vi "Split Registers by Direction.vi"(8 "error in":errorcluster, 11 "vi info":T1 {"RegisterMap"."Address" format="%.0x"}) -> (0 "error out":errorcluster, 2 "Controls":T8[](array[typedef]) {"Data Type" format="%.0x"}, 3 "Indicator":T8[](array[typedef]) {"Data Type" format="%.0x"})   [LabVIEW 2016, in "FPGA Addon System Explorer.lvlib"]
uses:
  FPGA Addon System Explorer.lvlib
  Shared/Register Information.ctl
  Shared/Data Type.ctl
  <vilib>/rvi/Bitfile/niFpgaBitfileStructure_VI.ctl
  <vilib>/rvi/Bitfile/nirviControlStructure.ctl
  <vilib>/rvi/Bitfile/nirviTypdefDescription.ctl
  <vilib>/rvi/Bitfile/nirviMechanicalAction.ctl
  <vilib>/rvi/Bitfile/nirviSubControlStructure.ctl
  <vilib>/rvi/Bitfile/nirviClusterElementControl.ctl
  <vilib>/picture/picture.llb/imagedata.ctl
  FPGA/Speciality IO/Types/PWM.Measure.Analog.Measurement.ctl
  FPGA/Speciality IO/Types/PWM.Measure.Digital.Measurement.ctl
  FPGA/Speciality IO/Types/PWM.Generate.Digital.Settings.ctl
  FPGA/Speciality IO/Types/PWM.Measure.Analog.Settings.ctl
  FPGA/Speciality IO/Types/PWM.Measure.Digital.Settings.ctl
  FPGA/Speciality IO/Types/Sine.Generate.Settings.ctl
  Shared/FPGA Addon Shared.lvlib
  FPGA/Speciality IO/Speciality FPGA IO.lvlib
  <vilib>/Utility/Data Type/NI_Data Type.lvlib
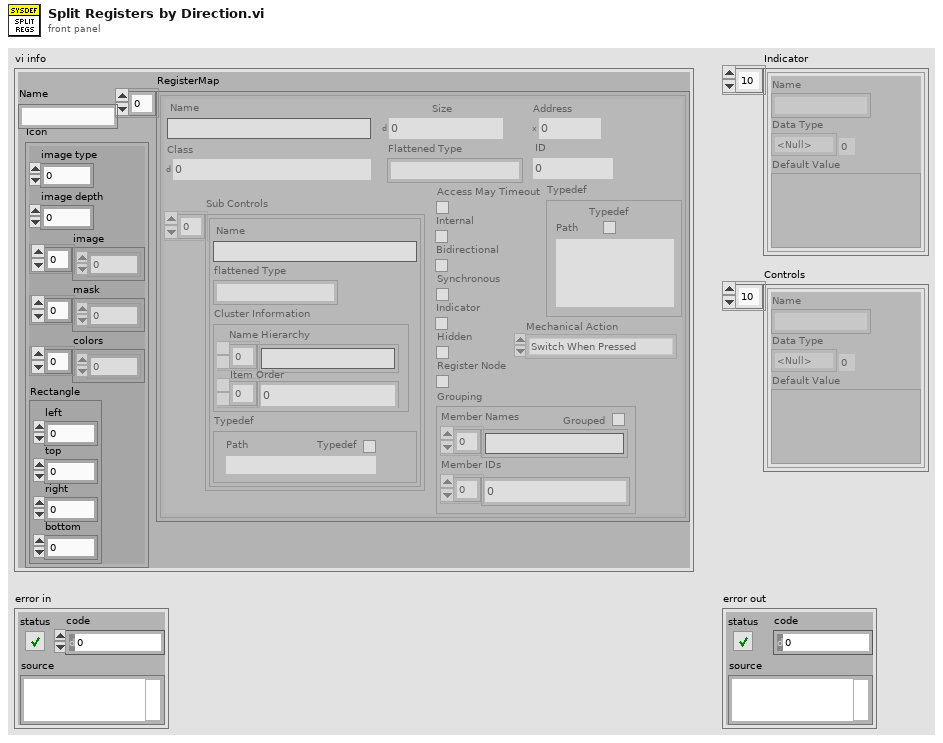
[diagram p1: front panel]
types:
  T1 = typedef "niFpgaBitfileStructure_VI.ctl" = cluster{"Name":string, "RegisterMap":T2[], "Icon":T7}
  T2 = typedef "nirviControlStructure.ctl" = cluster{"Name":string, "Hidden":bool, "Indicator":bool, "Flattened Type":string, "Grouping":cluster{"Grouped":bool, "Member Names":string[], "Member IDs":u32[]}, "Address":u32, "Size":u32, "Class":u32, "Internal":bool, "Typedef":T3, "ID":u32, "Bidirectional":bool, "Synchronous":bool, "Mechanical Action":T4, "Sub Controls":T5[], "Access May Timeout":bool, "Register Node":bool}
  T3 = typedef "nirviTypdefDescription.ctl" = cluster{"Typedef":bool, "Path":path}
  T4 = typedef "nirviMechanicalAction.ctl" = enum8{"Switch When Pressed", "Switch When Released", "Switch Until Released", "Latch When Pressed", "Latch When Released", "Latch Until Released"}
  T5 = typedef "nirviSubControlStructure.ctl" = cluster{"Name":string, "flattened Type":string, "Cluster Information":T6, "Typedef":T3}
  T6 = typedef "nirviClusterElementControl.ctl" = cluster{"Name Hierarchy":string[], "Item Order":u32[]}
  T7 = typedef "imagedata.ctl" = cluster{"image type":i32, "image depth":i32, "image":u8[], "mask":u8[], "colors":u32[], "Rectangle":cluster{"left":i16, "top":i16, "right":i16, "bottom":i16}}
  T8 = typedef "FPGA Addon Shared.lvlib/Register Information.ctl" = cluster{"Name":string, "Data Type":T9, "Default Value":variant}
  T9 = typedef "FPGA Addon Shared.lvlib/Data Type.ctl" = enum8{"<Null>", "I8", "I16", "I32", "I64", "U8", "U16", "U32", "U64", "SGL", "Boolean", "Analog PWM In Settings", "Analog PWM In", "Digital PWM In Settings", "Digital PWM In", "Digital PWM Out", "Sine Out", "FXP+/-24.5", "FXP+/-16.5", "FXP+/-32.8", "FXP+/-64.32", "FXP+/-16.7", "FXP+/-20.5"}
  T10 = typedef "Speciality FPGA IO.lvlib/PWM.Measure.Digital.Measurement.ctl" = cluster{"ACTIVE TICKS":u32, "INACTIVE TICKS":u32, "ACQ TICKS":u32}
  T11 = typedef "Speciality FPGA IO.lvlib/PWM.Measure.Analog.Measurement.ctl" = cluster{"ACTIVE TICKS":u32, "INACTIVE TICKS":u32, "ACQ TICKS":u32, "ACTIVE VOLTAGE":fxp<+/-,32,8>, "INACTIVE VOLTAGE":fxp<+/-,32,8>}
  T12 = typedef "Speciality FPGA IO.lvlib/Sine.Generate.Settings.ctl" = cluster{"AMP":fxp<+/-,32,8>, "OFFSET":fxp<+/-,32,8>, "PERIODS/TICKS":fxp<+,32,0>}
  T13 = typedef "Speciality FPGA IO.lvlib/PWM.Measure.Digital.Settings.ctl" = cluster{"ACTIVE EDGE":bool, "TIMEOUT":u32}
  T14 = typedef "Speciality FPGA IO.lvlib/PWM.Measure.Analog.Settings.ctl" = cluster{"ACTIVE EDGE":bool, "TIMEOUT":u32, "THRESHOLD":fxp<+/-,32,8>}
  T15 = typedef "Speciality FPGA IO.lvlib/PWM.Generate.Digital.Settings.ctl" = cluster{"ACTIVE EDGE":bool, "ACTIVE TICKS":u32, "INACTIVE TICKS":u32}
  T16 = typedef "NI_Data Type.lvlib/Data Type.ctl" = enum8{"Invalid Type", "Void", "I8", "I16", "I32", "I64", "U8", "U16", "U32", "U64", "Single Float", "Double Float", "Extended Float", "Single Complex", "Double Complex", "Extended Complex", "Enum U8", "Enum U16", "Enum U32", "Enum U64", "Single Float With Unit", "Double Float With Unit", "Extended Float With Unit", "Single Complex with Unit", "Double Complex with Unit", "Extended Complex with Unit", "Boolean", "String", "Path", "Picture", "Tag", "Array", "Cluster", "Variant", "LV Variant", "Waveform", "Timestamp", "Digital Waveform", "Digital Data", "ExpressData", "Refnum", "External Data", "VI", "Poly VI", "LabVIEW Class Instance", "Fixed Point"}
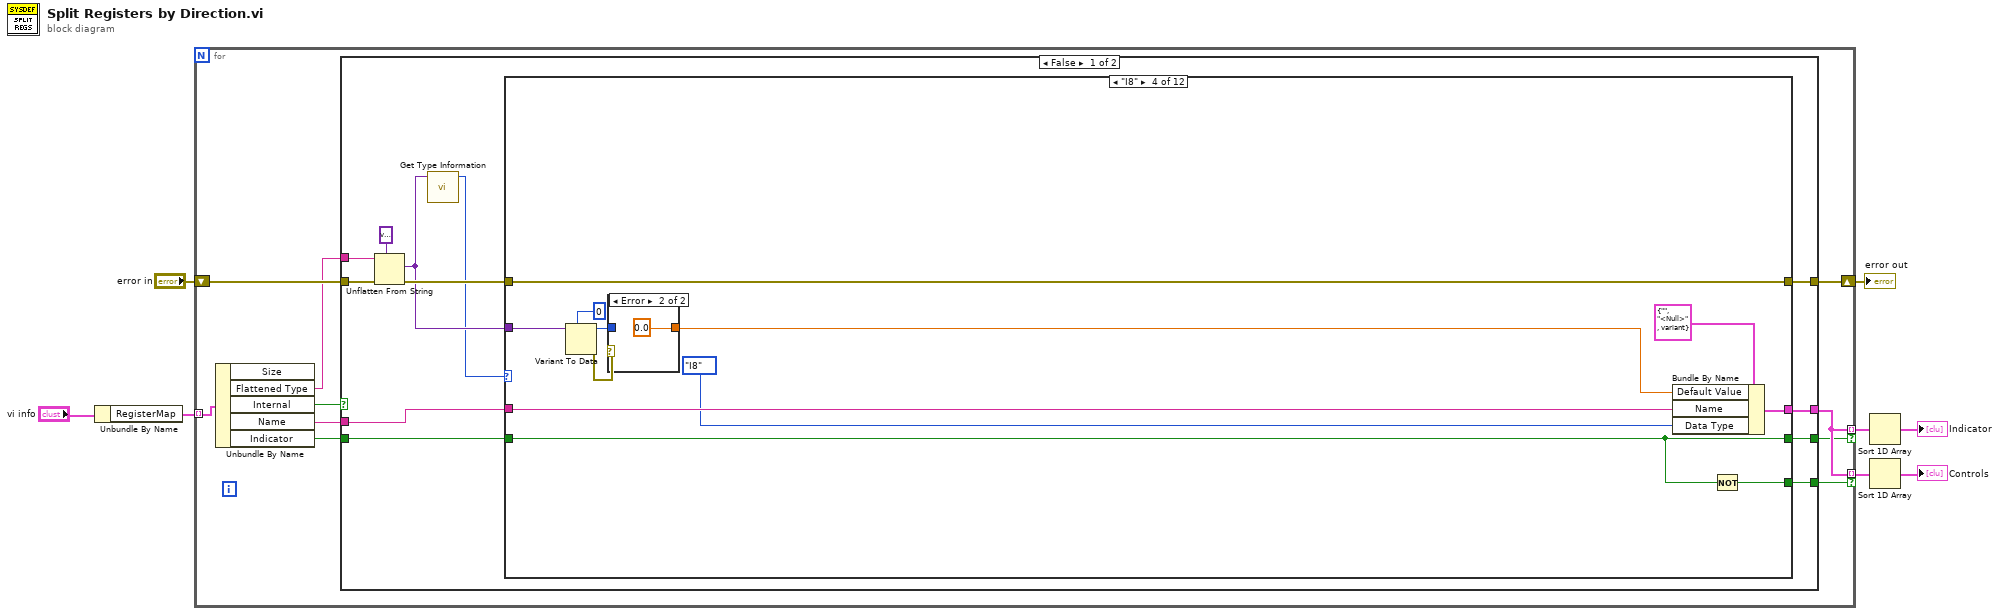
[diagram p0: block diagram]
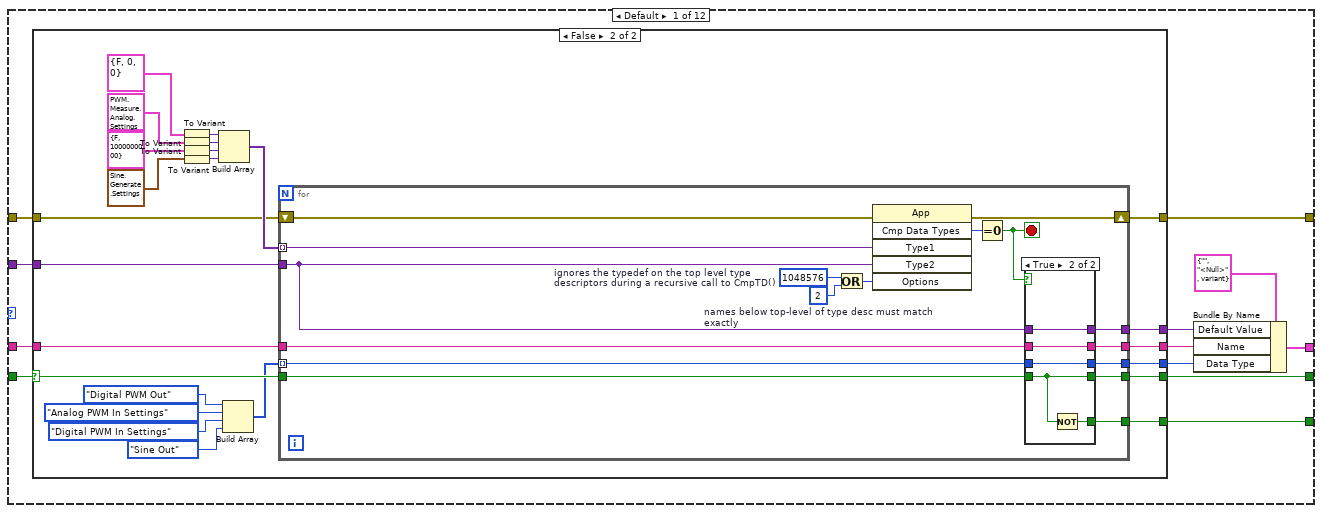
[diagram p2: hidden frame]
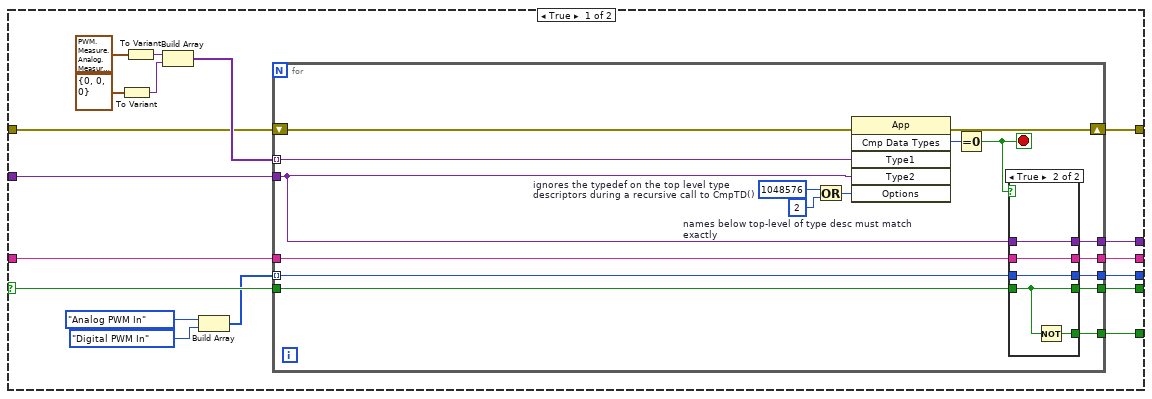
[diagram p3: hidden frame]
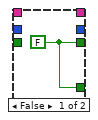
[diagram p4: hidden frame]
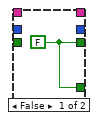
[diagram p5: hidden frame]
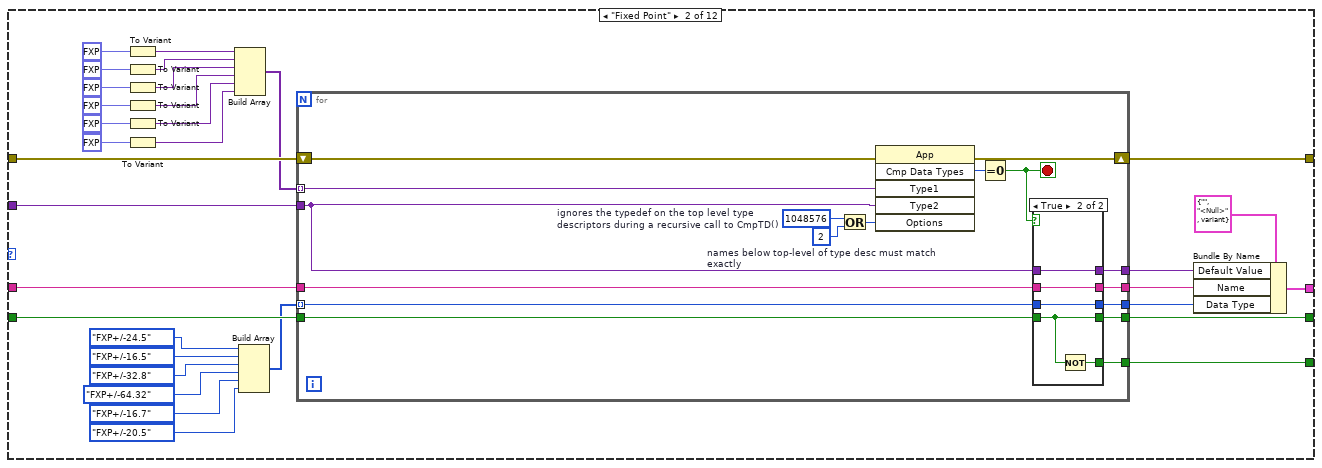
[diagram p6: hidden frame]
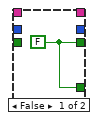
[diagram p7: hidden frame]
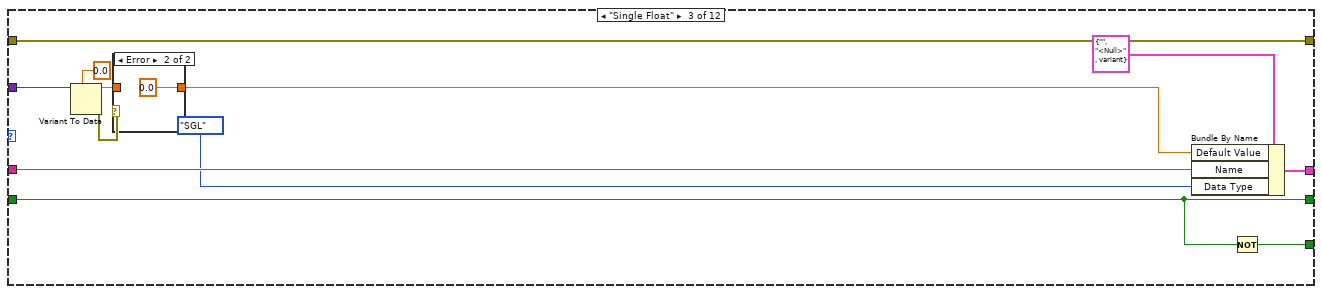
[diagram p8: hidden frame]
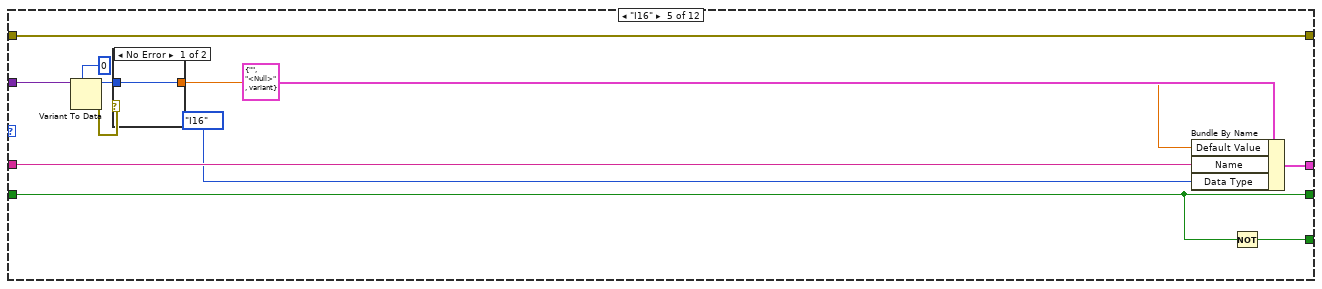
[diagram p11: hidden frame]
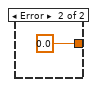
[diagram p12: hidden frame]
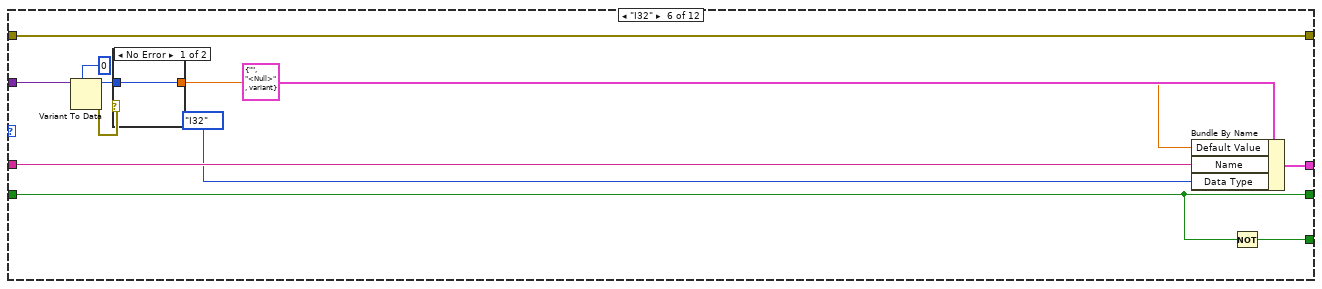
[diagram p13: hidden frame]
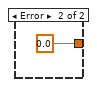
[diagram p14: hidden frame]
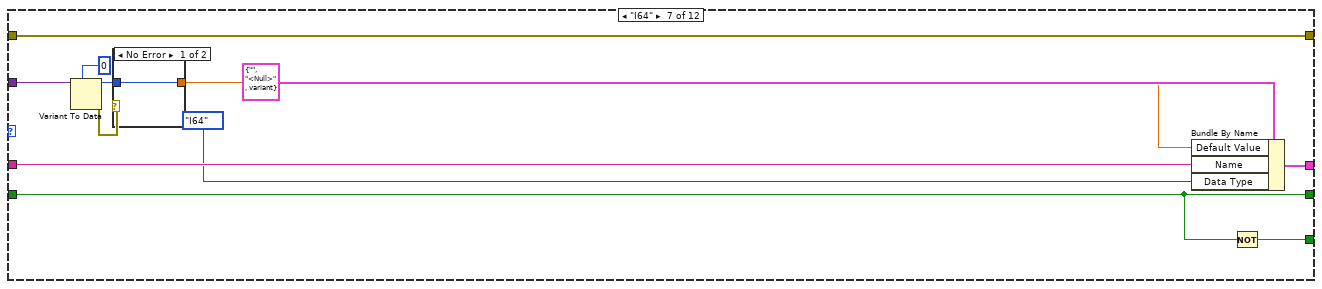
[diagram p15: hidden frame]
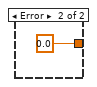
[diagram p16: hidden frame]
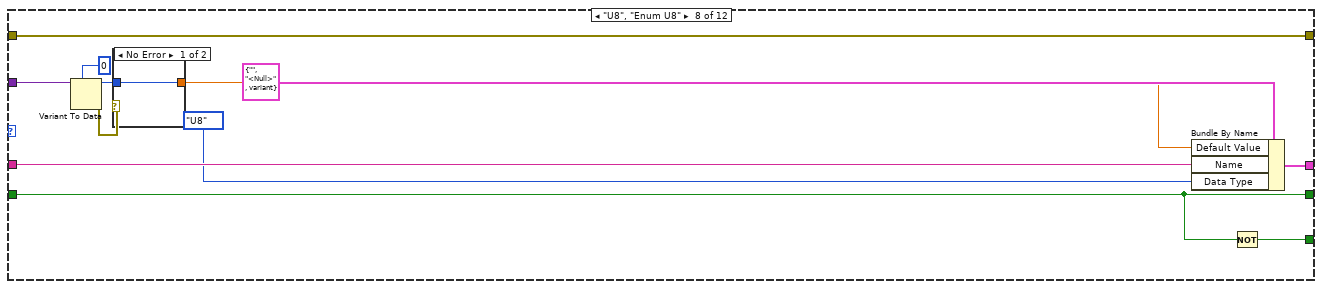
[diagram p17: hidden frame]
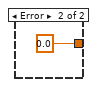
[diagram p18: hidden frame]
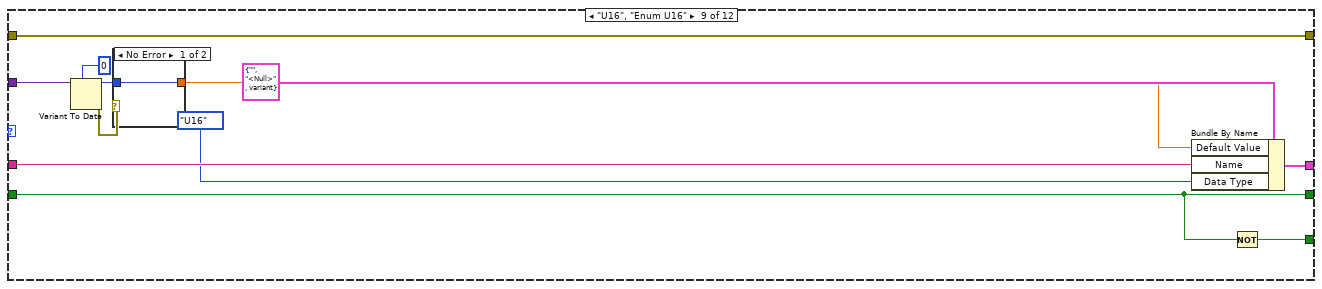
[diagram p19: hidden frame]
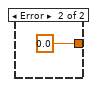
[diagram p20: hidden frame]
diagram:
  n1 = Unbundle By Name("vi info") -> ("RegisterMap"=w6:T2[])
  n2 = for {
    tunnel: w6 -> [w13] mode=indexing
    tunnel: [w18] -> w7 mode=indexing if=w17
    tunnel: [w18] -> w8 mode=indexing if=w16
    shift-right: [w15] -> w2
    shift-left: "error in" -> [w14]
    n3 = Unbundle By Name(w13) -> ("Flattened Type"=w9:string, "Internal"=w10:bool, "Name"=w11:string, "Indicator"=w12:bool)  [unwired: 1 out]
    n4 = case shown="False" w10 {
      tunnel: w11 -> [w30 _]
      tunnel: w12 -> [w29 _]
      tunnel: [w28 _] -> w18
      tunnel: [w27 w328] -> w17
      tunnel: [w26 w328] -> w16
      tunnel: w9 -> [w23 _]
      tunnel: [w25 w327] -> w15
      tunnel: w14 -> [w22 w327]
      frame False {
        n5 = Unflatten From String(type=variant ("Variant"), binary string=w23, error in (no error)=w22) -> (value=w20:variant, error out=w21:errorcluster)  [unwired: 3 out]
        n6 = call <vilib>:"Get Type Information.vi"("Variant"=w20) -> ("Type"=w19:T16)  [unwired: 6 in, 4 out]
        n7 = case shown="\"I8\"" w19 {
          tunnel: [w42 w162 w194 w208 w222 w236 w250 w264 w278 w292 w306 w320] -> w27
          tunnel: w29 -> [w37 w157 w194 w208 w222 w236 w250 w264 w278 w292 w306 w320]
          tunnel: w30 -> [w38 w158 w196 w210 w224 w238 w252 w266 w280 w294 w308 w322]
          tunnel: [w39 w159 w195 w209 w223 w237 w251 w265 w279 w293 w307 w321] -> w28
          tunnel: [w41 w161 w193 w207 w221 w235 w249 w263 w277 w291 w305 w319] -> w26
          tunnel: w20 -> [w36 w156 w192 w206 w220 w234 w248 w262 w276 w290 w304 w318]
          tunnel: [w32 w152 w186 w200 w214 w228 w242 w256 w270 w284 w298 w312] -> w25
          tunnel: w21 -> [w31 w151 w186 w200 w214 w228 w242 w256 w270 w284 w298 w312]
          frame Default {
            n8 = case shown="False" w37 {
              selector: w37 -> [w55 w103]
              tunnel: [w60 w107] -> w42
              tunnel: [w59 w106] -> w41
              tunnel: w38 -> [w58 w105]
              tunnel: w36 -> [w49 w99]
              tunnel: [w48 w98] -> w35
              tunnel: [w47 w97] -> w34
              tunnel: [w46 w96] -> w33
              tunnel: [w44 w87] -> w32
              tunnel: w31 -> [w43 w88]
              frame True {
                n9 = To Variant(anything=T10 {"ACTIVE TICKS"=0, "INACTIVE TICKS"=0, "ACQ TICKS"=0} ("Cached.Data")) -> (Variant=w53:variant)
                n10 = To Variant(anything=T11 {"ACTIVE TICKS"=0, "INACTIVE TICKS"=0, "ACQ TICKS"=0, "ACTIVE VOLTAGE"=0.0, "INACTIVE VOLTAGE"=0.0} ("Cached.Data")) -> (Variant=w54:variant)
                n11 = Build Array(w54, w53) -> (w50:variant[])
                n12 = Build Array(Data_Type."Analog PWM In" ("Data Type"), Data_Type."Digital PWM In" ("Data Type")) -> (w45:T9[])
                n13 = for {
                  tunnel: w49 -> [w64]
                  tunnel: [w75] -> w59
                  tunnel: w58 -> [w74]
                  tunnel: w50 -> [w66] mode=indexing
                  tunnel: [w73] -> w47
                  tunnel: [w72] -> w48
                  tunnel: [w71] -> w46
                  tunnel: w45 -> [w70] mode=indexing
                  tunnel: w55 -> [w77]
                  tunnel: [w76] -> w60
                  shift-right: [w61] -> w44
                  shift-left: w43 -> [w62]
                  stop <- w65 stop-if-true
                  w63 = 2  # names below top-level of type desc must match exactly
                  w68 = 1048576  # ignores the typedef on the top level type descriptors during a recursive call to CmpTD()
                  n14 = Or(x=w68, y=w63) -> (x .or. y?=w69:i32)
                  n15 = invoke class="App" method="Cmp Data Types"(error in=w62, "Type1"=w66, "Type2"=w64, "Options"=w69) -> (error out=w61:errorcluster, "Compare Data Types"=w67:i32)  [unwired: 2 in, 4 out]
                  n16 = Equal To 0?(x=w67) -> (x = 0?=w65:bool)
                  n17 = case shown="True" w65 {
                    tunnel: w77 -> [_ w83]
                    tunnel: [w78 w83] -> w76
                    tunnel: [w78 w82] -> w75
                    tunnel: w74 -> [_ w80]
                    tunnel: [_ w81] -> w73
                    tunnel: w64 -> [_ w81]
                    tunnel: [_ w80] -> w72
                    tunnel: [_ w79] -> w71
                    tunnel: w70 -> [_ w79]
                    frame False {
                      w78 = FALSE ("Boolean")
                    }
                    frame True {
                      n18 = Not(x=w83) -> (.not. x?=w82:bool)
                    }
                  }
                }
              }
              frame False {
                n19 = To Variant(anything=T15 {"ACTIVE EDGE"=FALSE, "ACTIVE TICKS"=0, "INACTIVE TICKS"=0} ("Channel.Settings")) -> (Variant=w102:variant)
                n20 = To Variant(anything=T14 {"ACTIVE EDGE"=FALSE, "TIMEOUT"=1000000000, "THRESHOLD"=3.0} ("Channel.Settings")) -> (Variant=w92:variant)
                n21 = To Variant(anything=T13 {"ACTIVE EDGE"=FALSE, "TIMEOUT"=1000000000} ("Channel.Settings")) -> (Variant=w91:variant)
                n22 = To Variant(anything=T12 {"AMP"=0.0, "OFFSET"=0.0, "PERIODS/TICKS"=0.0002500000409781933} ("Settings")) -> (Variant=w85:variant)
                n23 = Build Array(w102, w92, w91, w85) -> (w100:variant[])
                n24 = Build Array(Data_Type."Digital PWM Out" ("Data Type"), Data_Type."Analog PWM In Settings" ("Data Type"), Data_Type."Digital PWM In Settings" ("Data Type"), Data_Type."Sine Out" ("Data Type")) -> (w95:T9[])
                n25 = for {
                  tunnel: w99 -> [w113]
                  tunnel: [w122] -> w106
                  tunnel: w105 -> [w121]
                  tunnel: w100 -> [w112] mode=indexing
                  tunnel: [w120] -> w97
                  tunnel: [w119] -> w98
                  tunnel: [w118] -> w96
                  tunnel: w95 -> [w117] mode=indexing
                  tunnel: w103 -> [w124]
                  tunnel: [w123] -> w107
                  shift-right: [w108] -> w87
                  shift-left: w88 -> [w109]
                  stop <- w110 stop-if-true
                  w115 = 2  # names below top-level of type desc must match exactly
                  w114 = 1048576  # ignores the typedef on the top level type descriptors during a recursive call to CmpTD()
                  n26 = Or(x=w114, y=w115) -> (x .or. y?=w116:i32)
                  n27 = invoke class="App" method="Cmp Data Types"(error in=w109, "Type1"=w112, "Type2"=w113, "Options"=w116) -> (error out=w108:errorcluster, "Compare Data Types"=w111:i32)  [unwired: 2 in, 4 out]
                  n28 = Equal To 0?(x=w111) -> (x = 0?=w110:bool)
                  n29 = case shown="True" w110 {
                    tunnel: w124 -> [_ w130]
                    tunnel: [w125 w130] -> w123
                    tunnel: [w125 w129] -> w122
                    tunnel: w121 -> [_ w127]
                    tunnel: [_ w128] -> w120
                    tunnel: w113 -> [_ w128]
                    tunnel: [_ w127] -> w119
                    tunnel: [_ w126] -> w118
                    tunnel: w117 -> [_ w126]
                    frame False {
                      w125 = FALSE ("Boolean")
                    }
                    frame True {
                      n30 = Not(x=w130) -> (.not. x?=w129:bool)
                    }
                  }
                }
              }
            }
            n31 = Bundle By Name(cluster=T8 {"Name"="", "Data Type"=enum."<Null>", "Default Value"=variant(refnum<class> refnum)}, "Default Value"=w34, "Name"=w35, "Data Type"=w33) -> (w39:T8)
          }
          frame "Fixed Point" {
            n32 = To Variant(anything=fxp<+/-,24,5> 0.0 ("Numeric 1 In")) -> (Variant=w150:variant)
            n33 = To Variant(anything=fxp<+/-,16,5> 0.0 ("Numeric 2 In")) -> (Variant=w149:variant)
            n34 = To Variant(anything=fxp<+/-,32,8> 0.0 ("Numeric 3 In")) -> (Variant=w142:variant)
            n35 = To Variant(anything=fxp<+/-,64,32> 0.0 ("Numeric 4 In")) -> (Variant=w141:variant)
            n36 = To Variant(anything=fxp<+/-,16,7> 0.0 ("Numeric 4 In")) -> (Variant=w135:variant)
            n37 = To Variant(anything=fxp<+/-,20,5> 0.0 ("Numeric 4 In")) -> (Variant=w132:variant)
            n38 = Build Array(w150, w149, w142, w141, w135, w132) -> (w146:variant[])
            n39 = Build Array(Data_Type."FXP+/-24.5" ("Data Type"), Data_Type."FXP+/-16.5" ("Data Type"), Data_Type."FXP+/-32.8" ("Data Type"), Data_Type."FXP+/-64.32" ("Data Type"), Data_Type."FXP+/-16.7" ("Data Type"), Data_Type."FXP+/-20.5" ("Data Type")) -> (w145:T9[])
            n40 = for {
              tunnel: w156 -> [w166]
              tunnel: [w177] -> w161
              tunnel: w158 -> [w176]
              tunnel: w146 -> [w168] mode=indexing
              tunnel: [w175] -> w154
              tunnel: [w174] -> w155
              tunnel: [w173] -> w153
              tunnel: w145 -> [w172] mode=indexing
              tunnel: w157 -> [w179]
              tunnel: [w178] -> w162
              shift-right: [w163] -> w152
              shift-left: w151 -> [w164]
              stop <- w167 stop-if-true
              w165 = 2  # names below top-level of type desc must match exactly
              w170 = 1048576  # ignores the typedef on the top level type descriptors during a recursive call to CmpTD()
              n41 = Or(x=w170, y=w165) -> (x .or. y?=w171:i32)
              n42 = invoke class="App" method="Cmp Data Types"(error in=w164, "Type1"=w168, "Type2"=w166, "Options"=w171) -> (error out=w163:errorcluster, "Compare Data Types"=w169:i32)  [unwired: 2 in, 4 out]
              n43 = Equal To 0?(x=w169) -> (x = 0?=w167:bool)
              n44 = case shown="True" w167 {
                tunnel: w179 -> [_ w185]
                tunnel: [w180 w185] -> w178
                tunnel: [w180 w184] -> w177
                tunnel: w176 -> [_ w182]
                tunnel: [_ w183] -> w175
                tunnel: w166 -> [_ w183]
                tunnel: [_ w182] -> w174
                tunnel: [_ w181] -> w173
                tunnel: w172 -> [_ w181]
                frame False {
                  w180 = FALSE ("Boolean")
                }
                frame True {
                  n45 = Not(x=w185) -> (.not. x?=w184:bool)
                }
              }
            }
            n46 = Bundle By Name(cluster=T8 {"Name"="", "Data Type"=enum."<Null>", "Default Value"=variant(refnum<class> refnum)}, "Default Value"=w154, "Name"=w155, "Data Type"=w153) -> (w159:T8)
          }
          frame "Single Float" {
            n47 = Variant To Data(type=sgl 0.0, Variant=w192) -> (data=w188:sgl, error out=w190:errorcluster)  [unwired: 1 in]
            n48 = case shown="Error" w190 {
              tunnel: [w198 0.0] -> w189
              tunnel: w188 -> [w198 _]
              frame No Error {
              }
              frame Error {
              }
            }
            n49 = Bundle By Name(cluster=T8 {"Name"="", "Data Type"=enum."<Null>", "Default Value"=variant(refnum<class> refnum)}, "Default Value"=w189, "Name"=w196, "Data Type"=Data_Type."SGL") -> (w195:T8)
            n50 = Not(x=w194) -> (.not. x?=w193:bool)
          }
          frame "I8" {
            n51 = Variant To Data(type=i8 0, Variant=w206) -> (data=w202:i8, error out=w204:errorcluster)  [unwired: 1 in]
            n52 = case shown="Error" w204 {
              tunnel: [w212 0.0] -> w203
              tunnel: w202 -> [w212 _]
              frame No Error {
              }
              frame Error {
              }
            }
            n53 = Bundle By Name(cluster=T8 {"Name"="", "Data Type"=enum."<Null>", "Default Value"=variant(refnum<class> refnum)}, "Default Value"=w203, "Name"=w210, "Data Type"=Data_Type."I8") -> (w209:T8)
            n54 = Not(x=w208) -> (.not. x?=w207:bool)
          }
          frame "I16" {
            n55 = Variant To Data(type=i16 0, Variant=w220) -> (data=w216:i16, error out=w218:errorcluster)  [unwired: 1 in]
            n56 = case shown="No Error" w218 {
              tunnel: [w226 0.0] -> w217
              tunnel: w216 -> [w226 _]
              frame No Error {
              }
              frame Error {
              }
            }
            n57 = Bundle By Name(cluster=T8 {"Name"="", "Data Type"=enum."<Null>", "Default Value"=variant(refnum<class> refnum)}, "Default Value"=w217, "Name"=w224, "Data Type"=Data_Type."I16") -> (w223:T8)
            n58 = Not(x=w222) -> (.not. x?=w221:bool)
          }
          frame "I32" {
            n59 = Variant To Data(type=0, Variant=w234) -> (data=w230:i32, error out=w232:errorcluster)  [unwired: 1 in]
            n60 = case shown="No Error" w232 {
              tunnel: [w240 0.0] -> w231
              tunnel: w230 -> [w240 _]
              frame No Error {
              }
              frame Error {
              }
            }
            n61 = Bundle By Name(cluster=T8 {"Name"="", "Data Type"=enum."<Null>", "Default Value"=variant(refnum<class> refnum)}, "Default Value"=w231, "Name"=w238, "Data Type"=Data_Type."I32") -> (w237:T8)
            n62 = Not(x=w236) -> (.not. x?=w235:bool)
          }
          frame "I64" {
            n63 = Variant To Data(type=i64 0, Variant=w248) -> (data=w244:i64, error out=w246:errorcluster)  [unwired: 1 in]
            n64 = case shown="No Error" w246 {
              tunnel: [w254 0.0] -> w245
              tunnel: w244 -> [w254 _]
              frame No Error {
              }
              frame Error {
              }
            }
            n65 = Bundle By Name(cluster=T8 {"Name"="", "Data Type"=enum."<Null>", "Default Value"=variant(refnum<class> refnum)}, "Default Value"=w245, "Name"=w252, "Data Type"=Data_Type."I64") -> (w251:T8)
            n66 = Not(x=w250) -> (.not. x?=w249:bool)
          }
          frame "U8", "Enum U8" {
            n67 = Variant To Data(type=u8 0, Variant=w262) -> (data=w258:u8, error out=w260:errorcluster)  [unwired: 1 in]
            n68 = case shown="No Error" w260 {
              tunnel: [w268 0.0] -> w259
              tunnel: w258 -> [w268 _]
              frame No Error {
              }
              frame Error {
              }
            }
            n69 = Bundle By Name(cluster=T8 {"Name"="", "Data Type"=enum."<Null>", "Default Value"=variant(refnum<class> refnum)}, "Default Value"=w259, "Name"=w266, "Data Type"=Data_Type."U8") -> (w265:T8)
            n70 = Not(x=w264) -> (.not. x?=w263:bool)
          }
          frame "U16", "Enum U16" {
            n71 = Variant To Data(type=u16 0, Variant=w276) -> (data=w272:u16, error out=w274:errorcluster)  [unwired: 1 in]
            n72 = case shown="No Error" w274 {
              tunnel: [w282 0.0] -> w273
              tunnel: w272 -> [w282 _]
              frame No Error {
              }
              frame Error {
              }
            }
            n73 = Bundle By Name(cluster=T8 {"Name"="", "Data Type"=enum."<Null>", "Default Value"=variant(refnum<class> refnum)}, "Default Value"=w273, "Name"=w280, "Data Type"=Data_Type."U16") -> (w279:T8)
            n74 = Not(x=w278) -> (.not. x?=w277:bool)
          }
          frame "U32", "Enum U32" {
            n75 = Variant To Data(type=u32 0, Variant=w290) -> (data=w286:u32, error out=w288:errorcluster)  [unwired: 1 in]
            n76 = case shown="No Error" w288 {
              tunnel: [w296 0.0] -> w287
              tunnel: w286 -> [w296 _]
              frame No Error {
              }
              frame Error {
              }
            }
            n77 = Bundle By Name(cluster=T8 {"Name"="", "Data Type"=enum."<Null>", "Default Value"=variant(refnum<class> refnum)}, "Default Value"=w287, "Name"=w294, "Data Type"=Data_Type."U32") -> (w293:T8)
            n78 = Not(x=w292) -> (.not. x?=w291:bool)
          }
          frame "U64", "Enum U64" {
            n79 = Variant To Data(type=u64 0, Variant=w304) -> (data=w300:u64, error out=w302:errorcluster)  [unwired: 1 in]
            n80 = case shown="No Error" w302 {
              tunnel: [w310 0.0] -> w301
              tunnel: w300 -> [w310 _]
              frame No Error {
              }
              frame Error {
              }
            }
            n81 = Bundle By Name(cluster=T8 {"Name"="", "Data Type"=enum."<Null>", "Default Value"=variant(refnum<class> refnum)}, "Default Value"=w301, "Name"=w308, "Data Type"=Data_Type."U64") -> (w307:T8)
            n82 = Not(x=w306) -> (.not. x?=w305:bool)
          }
          frame "Boolean" {
            n83 = Variant To Data(type=FALSE, Variant=w318) -> (data=w314:bool, error out=w316:errorcluster)  [unwired: 1 in]
            n84 = case shown="No Error" w316 {
              tunnel: [w324 0.0] -> w315
              tunnel: w314 -> [w325 _]
              frame No Error {
                n85 = Boolean To (0,1)(Boolean=w325) -> (0, 1=w324:i16)
              }
              frame Error {
              }
            }
            n86 = Bundle By Name(cluster=T8 {"Name"="", "Data Type"=enum."<Null>", "Default Value"=variant(refnum<class> refnum)}, "Default Value"=w315, "Name"=w322, "Data Type"=Data_Type."Boolean") -> (w321:T8)
            n87 = Not(x=w320) -> (.not. x?=w319:bool)
          }
        }
      }
      frame True {
        w328 = FALSE ("Boolean")
      }
    }
  }
  "error out" <- w2
  n88 = Sort 1D Array(array=w7) -> (sorted array=→"Indicator":T8[])
  n89 = Sort 1D Array(array=w8) -> (sorted array=→"Controls":T8[])
